vi "To Waveform.vi"(8 "error in (no error)":errorcluster, 11 "Double in":refnum<class "Double.lvclass">) -> (0 "error out":errorcluster, 1 "Success?":bool, 3 "Waveform Array":waveform(dbl)[](array[waveform]))   [LabVIEW 2020, in "Data.lvlib" / "Double.lvclass"]
doc: "Interpret 'Data' as a Waveform Array. If impossible 'Success?' is set to FALSE"
uses:
  Double.lvclass
  Double.lvclass/Double.ctl
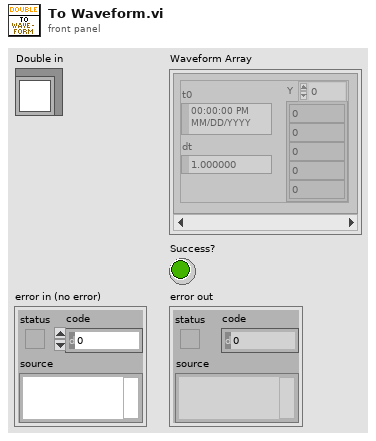
[diagram p1: front panel]
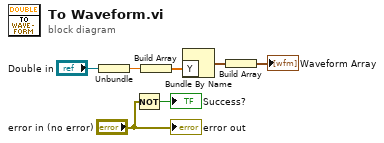
[diagram p0: block diagram]
diagram:
  n1 = Unbundle("Double in") -> (w6:dbl)
  n2 = Not(x="error in (no error)") -> (.not. x?=→"Success?":bool)
  n3 = Build Array(w6) -> (w4:dbl[])
  n4 = Bundle By Name("Y"=w4) -> (w7:waveform(dbl))  [unwired: 1 in]
  n5 = Build Array(w7) -> (→"Waveform Array":waveform(dbl)[])
  "error out" <- "error in (no error)"
